vi "Upload Segment.vi"(6 "Last Toggle Bit":bool, 7 "ICommunicate":refnum<class "ICommunicate.lvclass">, 8 "error in":errorcluster, 9 "Concetenated Value":u8[](array[numeric]), 10 "Service Data Object":refnum<class "Service Data Object.lvclass">, 11 "SDO Manager in":refnum<class "SDO Manager.lvclass">) -> (0 "error out":errorcluster, 1 "Concetenated Value out":u8[](array[numeric]), 2 "Success?":bool, 3 "SDO Manager out":refnum<class "SDO Manager.lvclass">)   [LabVIEW 2024]
uses:
  SDO Manager.lvclass/SDO Manager.ctl
  CANopen Response/CANopen Response Message.lvclass
  CANopen Request/CANopen Request Message.lvclass
  Service Data Object/Service Data Object.lvclass
  CANopen Message/CANopen Message.lvclass
  SDO Manager.lvclass
  HAL/Source/Interfaces/ICommunicate/ICommunicate.lvclass
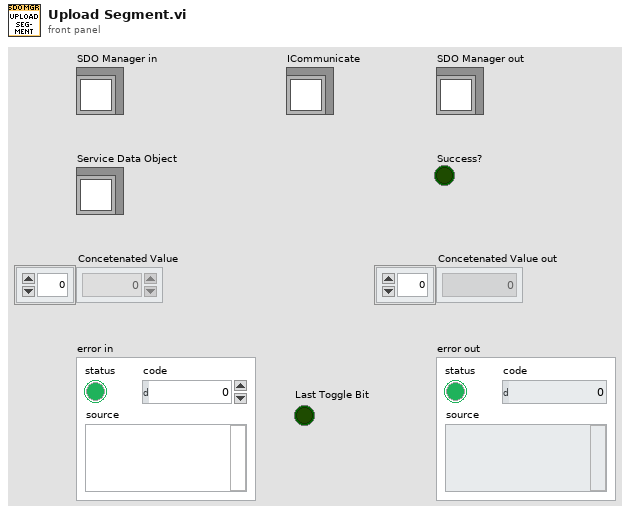
[diagram p1: front panel]
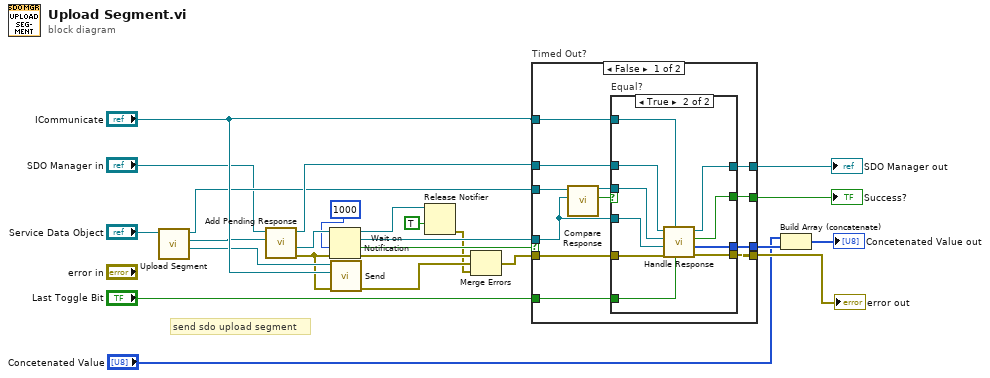
[diagram p0: block diagram]
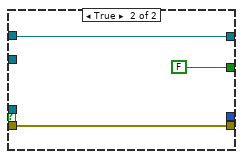
[diagram p3: hidden frame]
diagram:
  # "send sdo upload segment"
  n1 = call "Upload Segment.vi"("Service Data Object in"="Service Data Object") -> ("Request"=w16:refnum<class "CANopen Request Message.lvclass">, "Expected Response"=w17:refnum<class "CANopen Response Message.lvclass">, "Service Data Object out"=w20:refnum<class "Service Data Object.lvclass">)  [unwired: 8 in]
  n2 = call "Add Pending Response.vi"("Expected Response"=w17, "reference in"="SDO Manager in") -> ("Error Out"=w10:errorcluster, "Response Notifier out"=w19:refnum<notifier>, "reference out"=w22:refnum<class "SDO Manager.lvclass">)  [unwired: 7 in]
  n3 = Wait on Notification(notifier=w19, timeout in ms (-1)=1000, error in (no error)=w10) -> (notifier out=w2:refnum<notifier>, notification=w7:refnum<class "CANopen Response Message.lvclass">, timed out?=w6:bool, error out=w8:errorcluster)  [unwired: 1 in]
  n4 = call "Send.vi"("error in"=w10, "ICommunicate"="ICommunicate", "CANopen Message in"=w16) -> ("error out"=w4:errorcluster)  [unwired: 7 in, 1 out]
  n5 = Release Notifier(notifier=w2, force destroy? (F)=TRUE) -> (error out=w1:errorcluster)  [unwired: 1 in, 2 out]
  n6 = Merge Errors(w8, w4, w1) -> (w5:errorcluster)
  n7 = case "Timed Out?" shown="False" w6 {
    tunnel: w5 -> [w26 w53]
    tunnel: [w36 w53] -> w24
    tunnel: w7 -> [w34 _]
    tunnel: w20 -> [w37 _]
    tunnel: [w30 FALSE ("Equal?")] -> w25
    tunnel: [w35 w51] -> w23
    tunnel: "ICommunicate" -> [w32 _]
    tunnel: w22 -> [w31 w51]
    tunnel: [w29 _] -> w13
    tunnel: "Last Toggle Bit" -> [w27 _]
    frame False {
      n8 = call "Compare Response.vi"("Actual"=w34, "Service Data Object"=w37) -> ("Equal?"=w28:bool, "Service Data Object out"=w33:refnum<class "Service Data Object.lvclass">)  [unwired: 8 in]
      n9 = case "Equal?" shown="True" w28 {
        selector: w28 -> [w38 _]
        tunnel: w26 -> [w39 w50]
        tunnel: [w39 w49] -> w36
        tunnel: [w40 w48] -> w35
        tunnel: w34 -> [_ w47]
        tunnel: w33 -> [_ w46]
        tunnel: w32 -> [_ w45]
        tunnel: w31 -> [w40 w44]
        tunnel: [w38 w43] -> w30
        tunnel: [_ w42] -> w29
        tunnel: w27 -> [_ w41]
        frame False {
        }
        frame True {
          n10 = call "Handle Response.vi"("Last Toggle-Bit"=w41, "ICommunicate"=w45, "Error In"=w50, "Response"=w47, "Service Data Object"=w46, "reference in"=w44) -> ("Error Out"=w49:errorcluster, "Value"=w42:u8[], "Success?"=w43:bool, "reference out"=w48:refnum<class "SDO Manager.lvclass">)  [unwired: 2 in]
        }
      }
    }
    frame True {
    }
  }
  "Success?" <- w25
  "error out" <- w24
  "SDO Manager out" <- w23
  n11 = Build Array (concatenate)("Concetenated Value", w13) -> (→"Concetenated Value out":u8[])
